vi "Get Subpanel Ref.vi"(8 "error in (no error)":errorcluster, 11 "Optimiser SBlock in":refnum<class "Optimiser SBlock.lvclass">) -> (0 "error out":errorcluster, 2 "vi reference":refnum<vi>, 3 "Optimiser SBlock out":refnum<class "Optimiser SBlock.lvclass">)   [LabVIEW 2020, in "TALOS.lvlib" / "Run Utilities.lvlib" / "Optimiser SBlock.lvclass"]
uses:
  Optimiser SBlock.lvclass
  Optimiser SBlock.lvclass/Optimiser SBlock.ctl
  Optimiser Mode Panel.vi
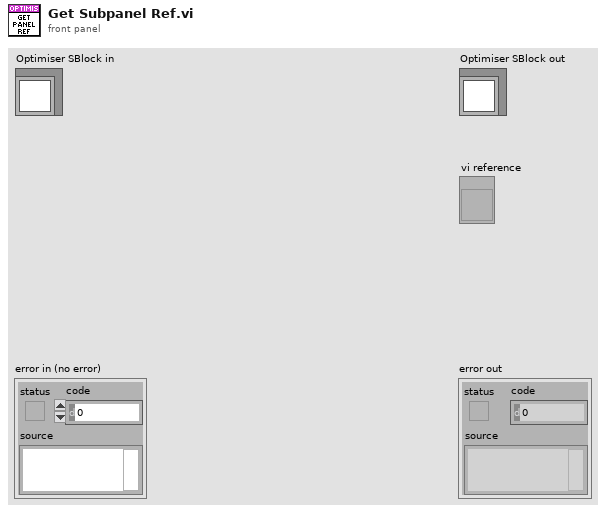
[diagram p1: front panel]
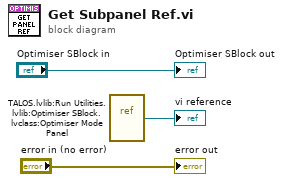
[diagram p0: block diagram]
diagram:
  n1 = vi-ref "TALOS.lvlib:Run Utilities.lvlib:Optimiser SBlock.lvclass:Optimiser Mode Panel.vi"() -> (→"vi reference":refnum<vi>)
  "error out" <- "error in (no error)"
  "Optimiser SBlock out" <- "Optimiser SBlock in"
